vi "Validate VAL SW.vi"() -> ()   [LabVIEW 2023, in "GUI.lvlib" / "Diagnostic.lvlib" / "VAL_SW_Testing.lvlib"]
uses:
  VAL_SW_Testing.lvlib
  HardwareAbstractionLayer_LVOOP/CAN/CAN Lib/CAN_class/Ctrls/CAN Init Ctrl.ctl
  <vilib>/xnet/xnet.llb/XNET Control Scope.ctl
  Ctrls/refresh.ctl
  Ctrls/stop.ctl
  Ctrls/File Paths.ctl
  HardwareAbstractionLayer_LVOOP/CAN/CAN Application Protocols/STP Protocol_class/Ctrls/STP CMD.ctl
  Ctrls/fwd.ctl
  Ctrls/refresh_sqr.ctl
  Ctrls/start.ctl
  HardwareAbstractionLayer_LVOOP/CAN/CAN Lib/Control/CAN Table.ctl
  HardwareAbstractionLayer_LVOOP/CAN/CAN Application Protocols/STP Protocol_class/Ctrls/STP Input Data.ctl
  HardwareAbstractionLayer_LVOOP/Database/SQL Public VI/Control/DB Options.ctl
  <vilib>/Utility/file.llb/Write Delimited Spreadsheet (string).vi
  <userlib>/_OpenG.lib/appcontrol/appcontrol.llb/openg_application_control.lvlib
  HardwareAbstractionLayer_LVOOP/CAN/CAN Application Protocols/STP Protocol_class/STP Protocol.lvclass
  HardwareAbstractionLayer_LVOOP/Database/Database.lvclass
  HardwareAbstractionLayer_LVOOP/CAN/CAN Lib/CAN_class/CAN.lvclass
  Teststand Steptypes/LTT_TeststandSteptypes.lvlib
  HardwareAbstractionLayer_LVOOP/CAN/CAN Lib/CAN HAL Lib.lvlib
panel:
  in  "Stop Button":T1
  in  "Tab Control":T2(tab)
  out "Response Data VAL SW":u8[](array[numeric]) caption="Data" format="%.0x"
  out "Request Timeout_mode":bool caption="Request Timeout?"
  out "+ve Response_Mode":bool caption="+ve Response?"
  in  "Latest_Irms":T3
  out "Irms":cluster{"Numeric 3":dbl, "Numeric 3":dbl}(knob)={"Numeric 3"=0.0, "Numeric 3"=30.81036768238346} scale=0.15..250.0
  in  "Stop Mode":T1
  out "Time Elapsed(Sec)":dbl format="%#.3g"
  in  "Start Mode":T4
  in  "Select Mode":u16(ring)=10 items=["Mode 1: eDCU ON / eMOTOR OFF"=1, "Mode 2: WMTC Pattern 1"=2, "Mode 3: WMTC Pattern 2"=3, "Mode 4: WMTC Pattern 3"=4, "Mode 5: WMTC Pattern 4"=5, "Mode 6: WMTC Pattern 5"=6, "Mode 7: WMTC Pattern 6"=7, "Mode 8: Worst case 1&3"=8, "Mode 9: Full power"=9, " Mode 10: Peak power (Worst case 1)"=10, "Mode 11 : Acceleration (Worst case 3)"=11, "Mode 12 : 1A RMS Continuous"=12, "Mode 13 : 5A RMS Continuous"=13, "Mode 14 : 70A RMS Continuous"=14]
  in  "VAL_Version":T3
  in  "TSW_Version":T3
  out "VAL SW Version":string
  out "TSW Version":string
  in  "Export":bool
  out "Request Timeout? Frame":bool caption="Request Timeout?"
  out "+ve Response? Frame":bool caption="+ve Response?"
  in  "Data Source":enum16{"CSV File", "CAN"}(ring)=enum."CAN"
  out "Datasize(Bytes)":i32
  out "Frame Data":u8[](array[numeric])
  in  "Frame Type":enum16{"FE Frame", "FF Frame"}(ring)
  in  "FE FF Refresh":T5
  in  "Raw_Data?":bool
  in  "Frame Detail":i32(listbox)
  out "Request Timeout?":bool
  out "ResponseData(ASCII)":string
  in  "Send CMD":T6
  out "+ve Response?":bool
  out "Response Data":u8[](array[numeric]) format="%.0x"
  in  "Write Data":u8[](array[numeric]) format="%.0x"
  in  "CMD":T7=130 items=["TSW_VERSION(130)"=130, "WAIT_EVENT(132)"=132, "SEQUENCER(133)"=133, "TSW_RESET(150)"=150, "CONFIG_ECU(151)"=151, "TEST_CORE (152)"=152, "TEST_WATCHDOG (153)"=153, "TEST_MONITORING (154)"=154, "READ_MEMORY (162)"=162, "WRITE_ERASE_MEMORY (164)"=164, "COMM_EXTERNAL (190)"=190, "COMM_INTERNAL (195)"=195, "GET_ANALOG_INPUT (210)"=210, "GET_DIGITAL_INPUT (211)"=211, "GET_FREQUENCY_INPUT (212)"=212, "TEST_INPUT_STRUCTURE (214)"=214, "GENERATE_OUTPUT_SIGNAL (220)"=220, "GENERATE_SYNCHRONIZED_OUTPUT_SIGNALS (221)"=221, "eDCU_Specific (250)"=250]
  in  "Echo?":bool
  in  "Log CAN Data":bool=TRUE
  in  "Timeout(Sec)":dbl=5.0
  in  "Config File Path":T8
  in  "CAN Init Data":T9={"XNET Interface"="CAN3", "Baud Rate"=1000000, "CAN:Termination"=0, "Echo Transmit?"=FALSE, "scope (normal)"=0} {"scope (normal)" items=["Normal", "Session Only", "Interface Only", "Session Only Blocking"]; "CAN:Termination" items=["Off", "On"]; "Baud Rate" format="%.0p"}
  in  "XNET Interface":refnum<k21>="CAN2"
  in  "CAN View Table":T11=-1
  # "Latest RMS Current(Amps)"
  # "SW Version"
  # "VAL Modes"
  # "Min"
  # "Max"
  # "Response"
  # "Request"
  # "Response"
  # "CAN Config"
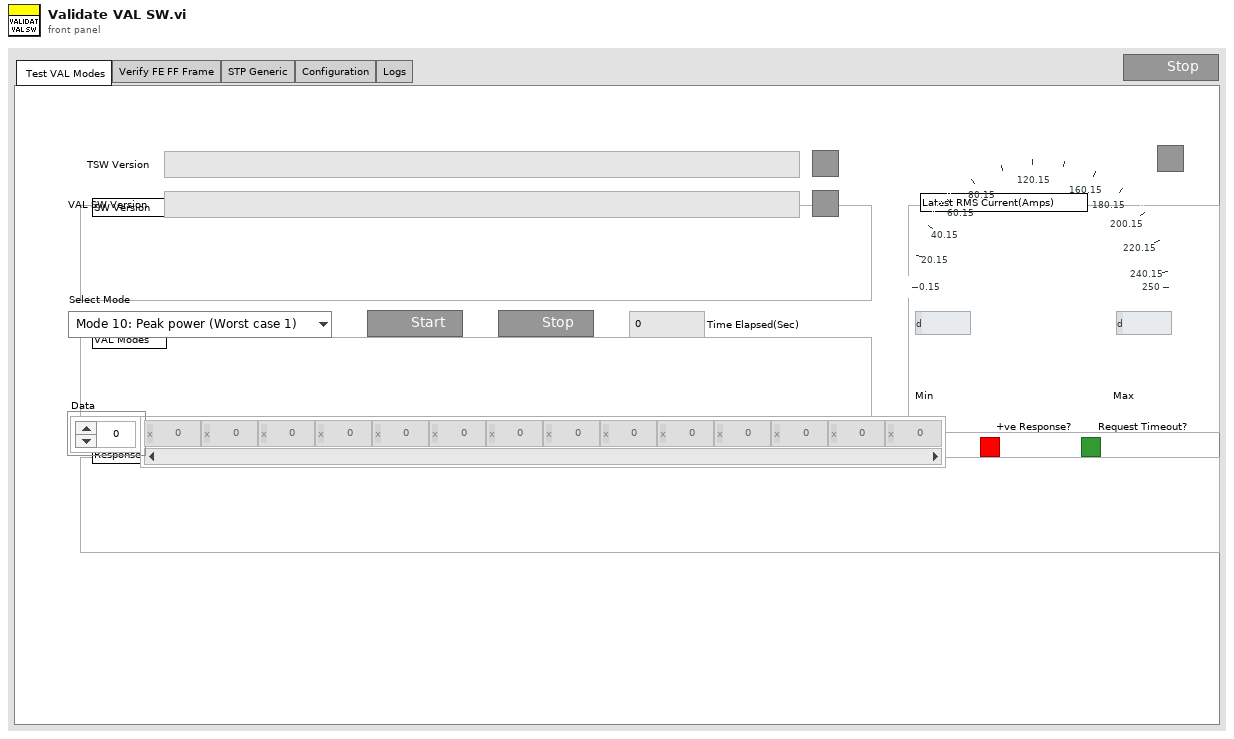
[diagram p1: front panel]
types:
  T1 = typedef "GUI.lvlib/Diagnostic.lvlib/VAL_SW_Testing.lvlib/stop.ctl" = bool
  T2 = enum32{" Test VAL Modes", "Verify FE FF Frame", "STP Generic", "Configuration", "Logs"}
  T3 = typedef "GUI.lvlib/Diagnostic.lvlib/VAL_SW_Testing.lvlib/refresh_sqr.ctl" = bool
  T4 = typedef "GUI.lvlib/Diagnostic.lvlib/VAL_SW_Testing.lvlib/start.ctl" = bool
  T5 = typedef "GUI.lvlib/Diagnostic.lvlib/VAL_SW_Testing.lvlib/refresh.ctl" = bool
  T6 = typedef "GUI.lvlib/Diagnostic.lvlib/VAL_SW_Testing.lvlib/fwd.ctl" = bool
  T7 = typedef "HardwareAbstractionLayer_LVOOP.lvlib/CAN Application Protocols Lib.lvlib/STP Protocol.lvclass/STP CMD.ctl" = u8
  T8 = typedef "GUI.lvlib/Diagnostic.lvlib/VAL_SW_Testing.lvlib/File Paths.ctl" = cluster{"FE_FF_Data File":path, "FE_Frame_Details_File":path, "FF_Frame_Details_File":path}
  T9 = typedef "HardwareAbstractionLayer_LVOOP.lvlib/CAN HAL Lib.lvlib/CAN.lvclass/CAN Init Ctrl.ctl" = cluster{"XNET Interface":refnum<k21>, "Baud Rate":u64, "CAN:Termination":u32, "Echo Transmit?":bool, "scope (normal)":T10}
  T10 = typedef "XNET Control Scope.ctl" = u32
  T11 = typedef "HardwareAbstractionLayer_LVOOP.lvlib/CAN HAL Lib.lvlib/CAN Table.ctl" = i32
  T12 = typedef "HardwareAbstractionLayer_LVOOP.lvlib/Database.lvclass/DB Options.ctl" = enum16{"Init", "Select Data", "Insert Data", "Update Data", "Delete Data", "Execute Query", "Create Schema", "Create Table", "List Tables", "List Columns", "Close"}
  T13 = typedef "HardwareAbstractionLayer_LVOOP.lvlib/CAN Application Protocols Lib.lvlib/STP Protocol.lvclass/STP Input Data.ctl" = cluster{"TxID":u32, "RxID":u32, "CMD":T7, "RQ Data":u8[], "+veResponseCode":u8, "ResponseTimeout (S)":dbl}
  T14 = enum16{"StartTimer", "ReadTimer", "StopTimer", "Init"}
  T15 = enum32{" Test VAL Modes", "Verify FE FF Frame", "STP Generic", "Configuration"}
  T16 = cluster{"Data Source":enum16{"CSV File", "CAN"}, "Frame Type":enum16{"FE Frame", "FF Frame"}, "Raw_Data?":bool, "Config File Path":T8, "CAN Init Data":T9, "ResponseTimeout (S)":dbl}
  T17 = typedef "HardwareAbstractionLayer_LVOOP.lvlib/CAN Application Protocols Lib.lvlib/STP Protocol.lvclass/STP Output Data.ctl" = cluster{"ResponseData":u8[], "ResponseData(ASCII)":string, "PositiveResponse?":bool, "STP Error":T18}
  T18 = typedef "HardwareAbstractionLayer_LVOOP.lvlib/CAN Application Protocols Lib.lvlib/STP Protocol.lvclass/STP Error Cluster.ctl" = cluster{"Status":bool, "Code":u8, "Error":string, "Description":string}
  T19 = cluster{"Frame Data":u8[], "Raw Data":u64[], "Signal Values":string[], "Datasize(Bytes)":i32}
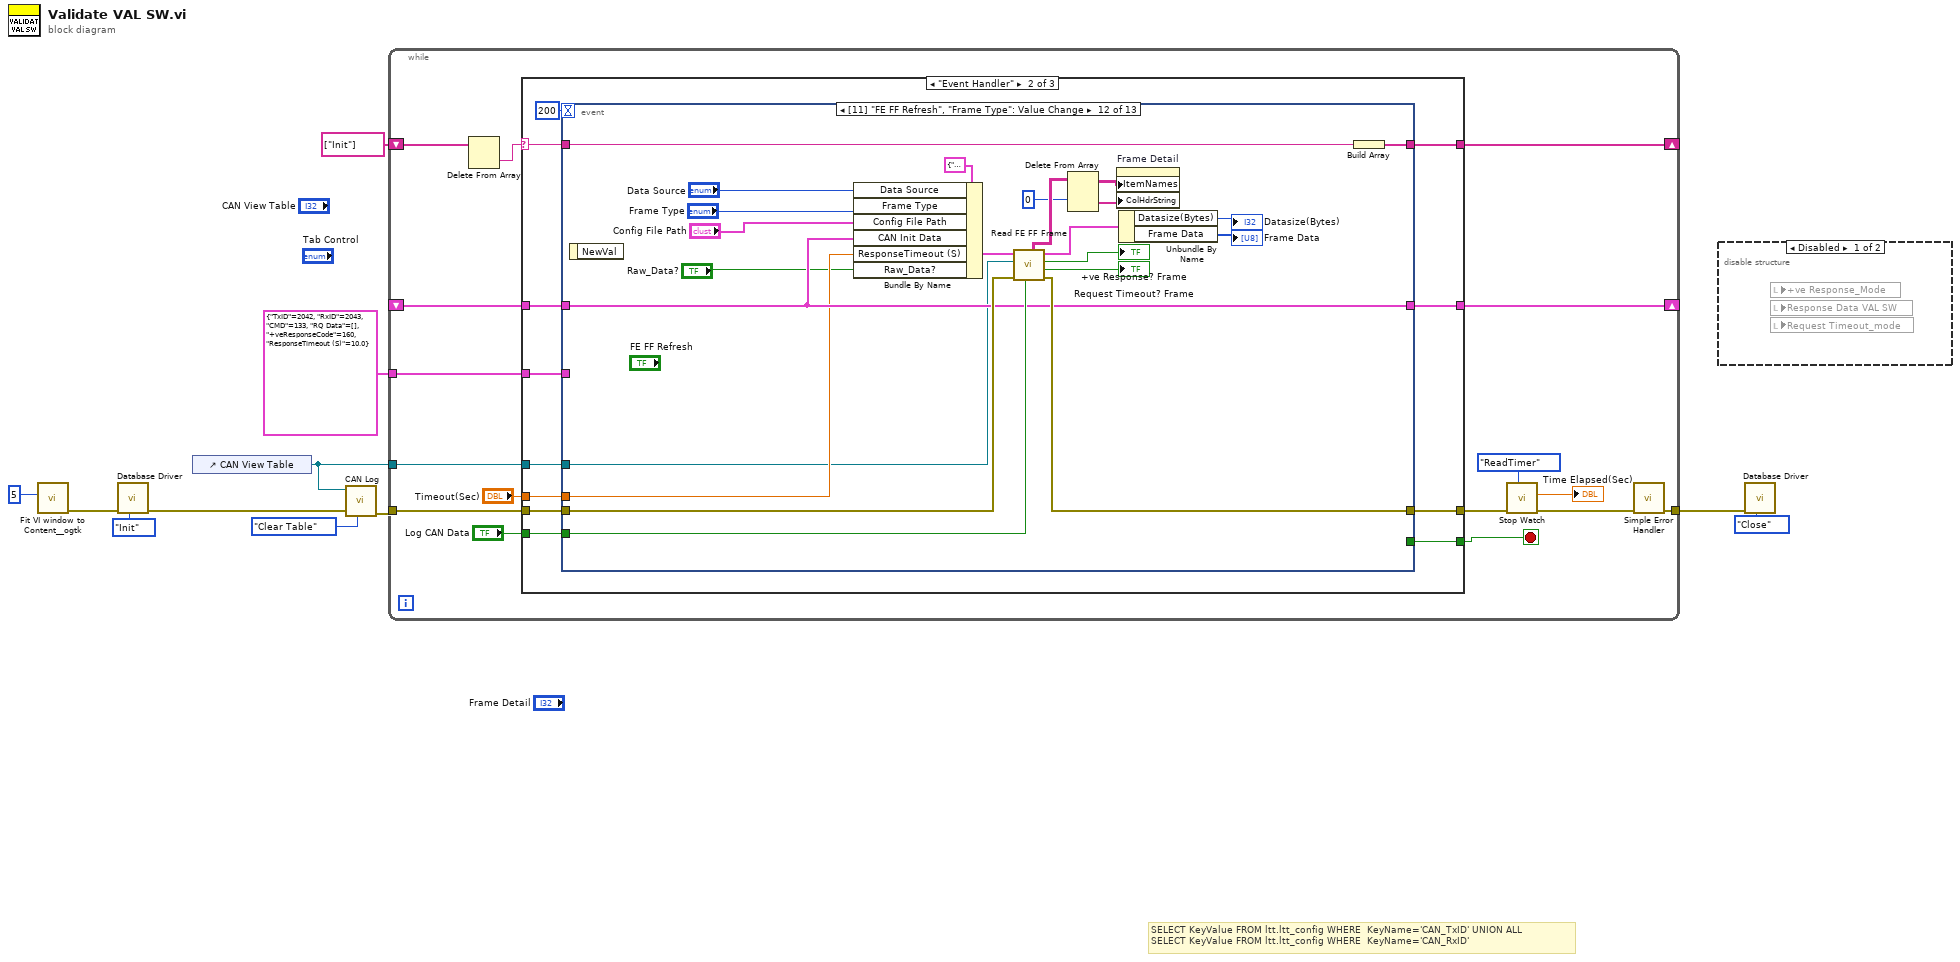
[diagram p0: block diagram]
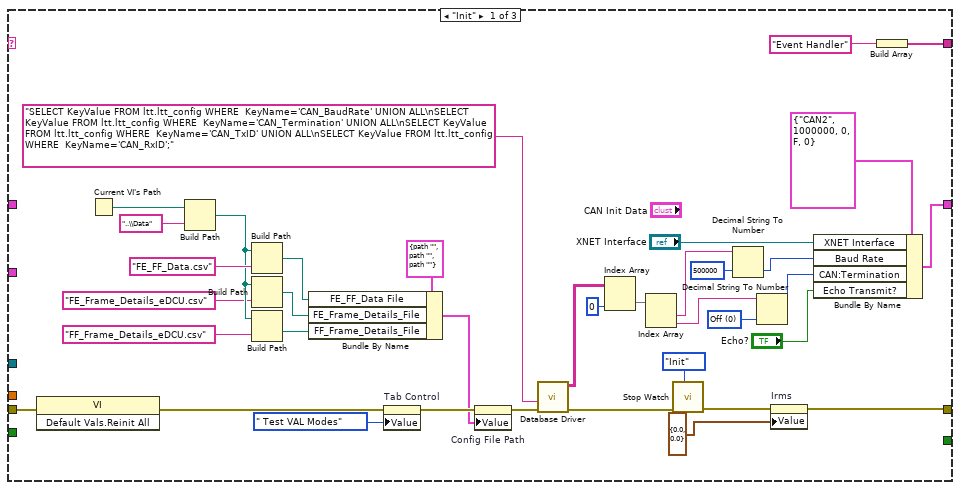
[diagram p3: hidden frame]
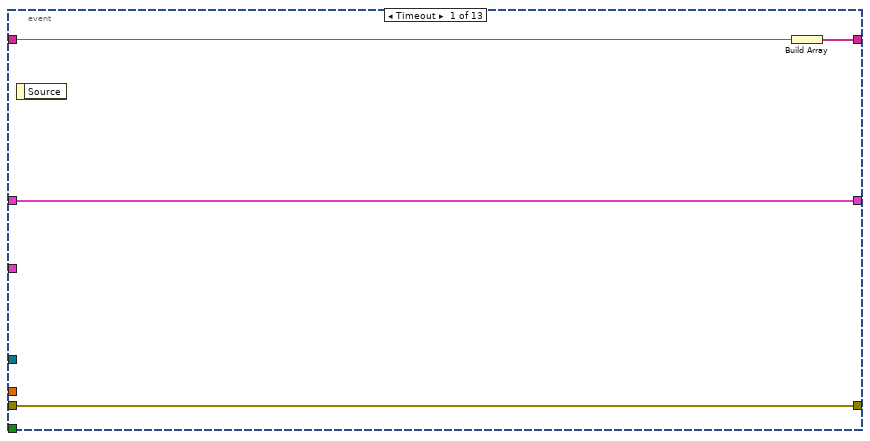
[diagram p4: hidden frame]
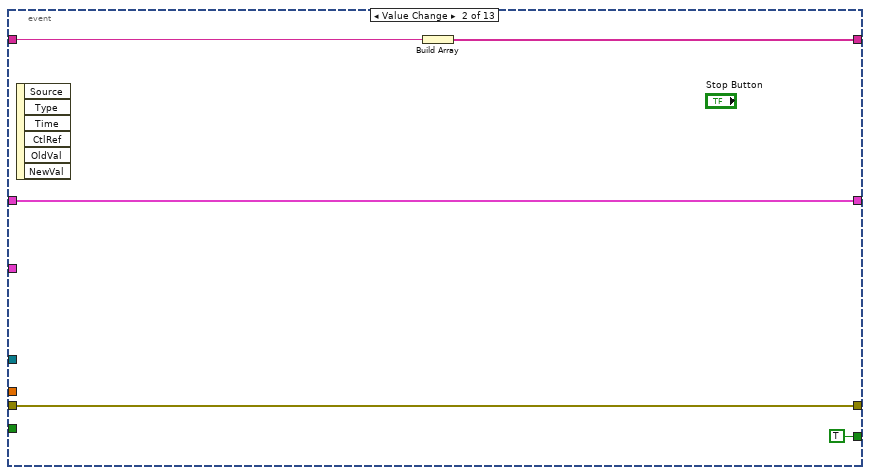
[diagram p5: hidden frame]
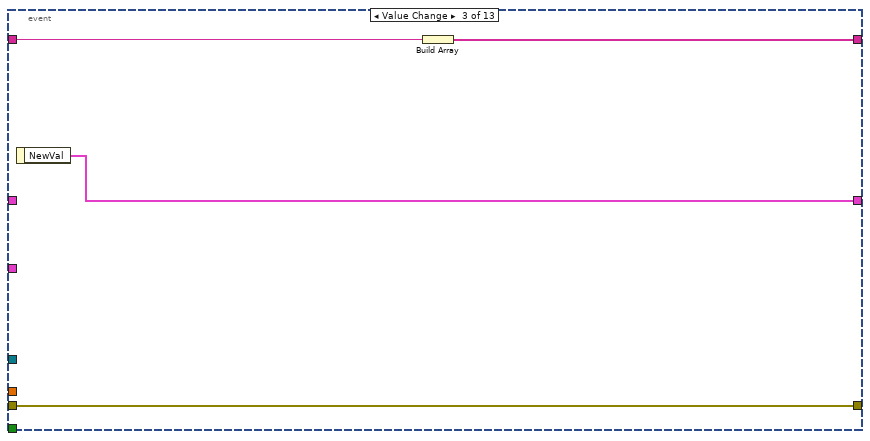
[diagram p6: hidden frame]
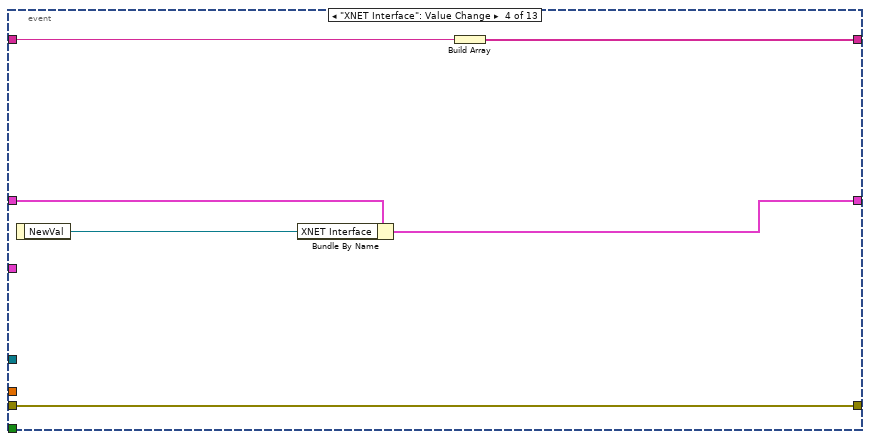
[diagram p7: hidden frame]
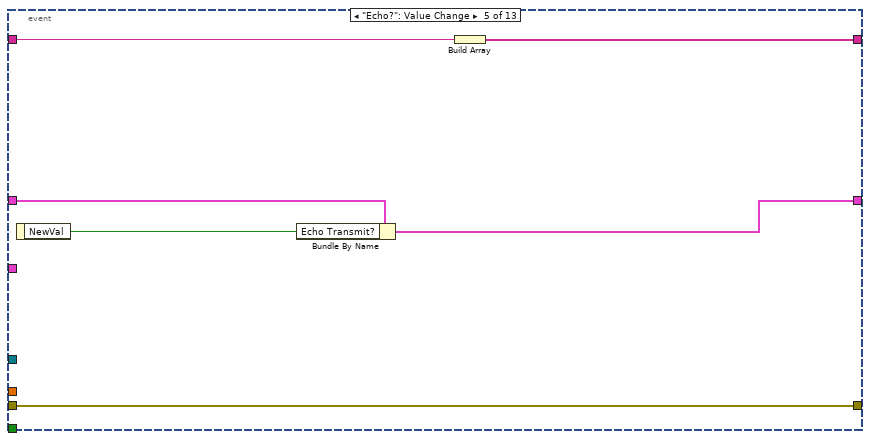
[diagram p8: hidden frame]
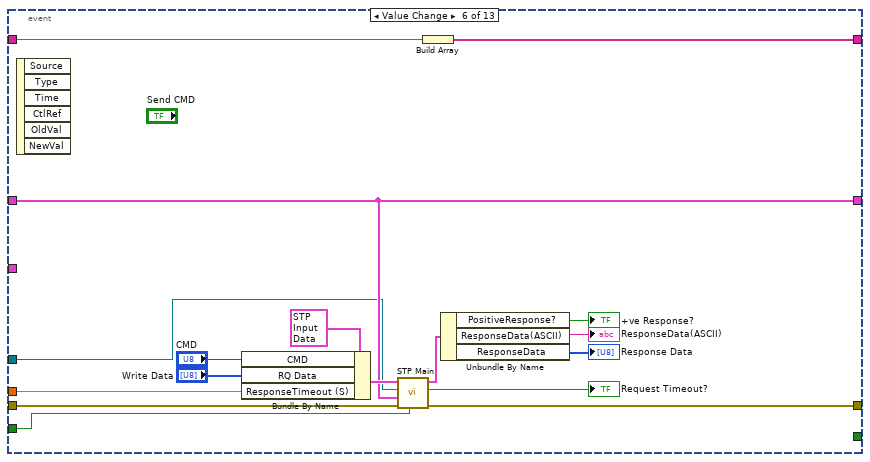
[diagram p9: hidden frame]
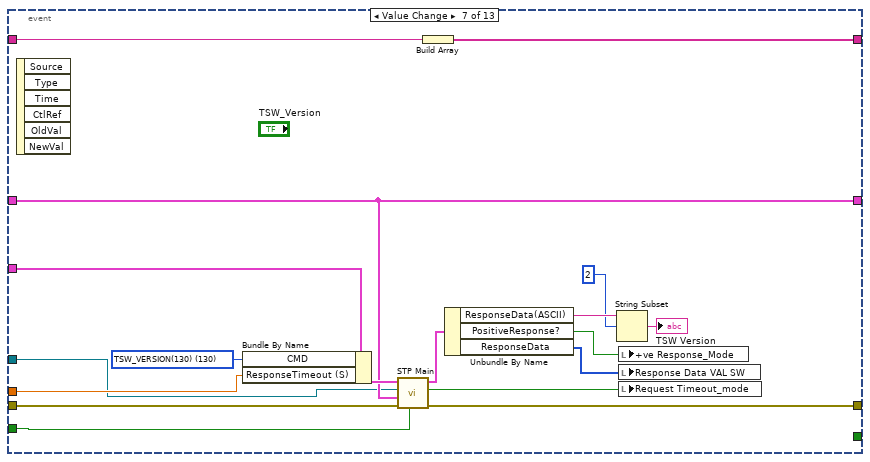
[diagram p10: hidden frame]
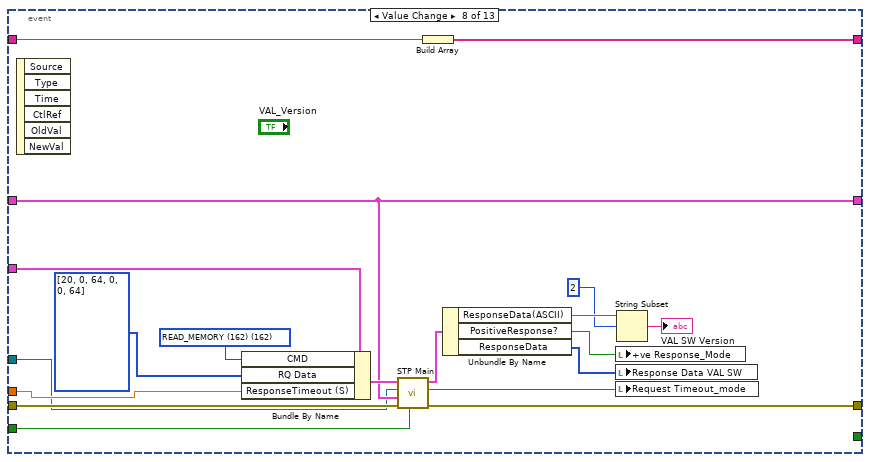
[diagram p11: hidden frame]
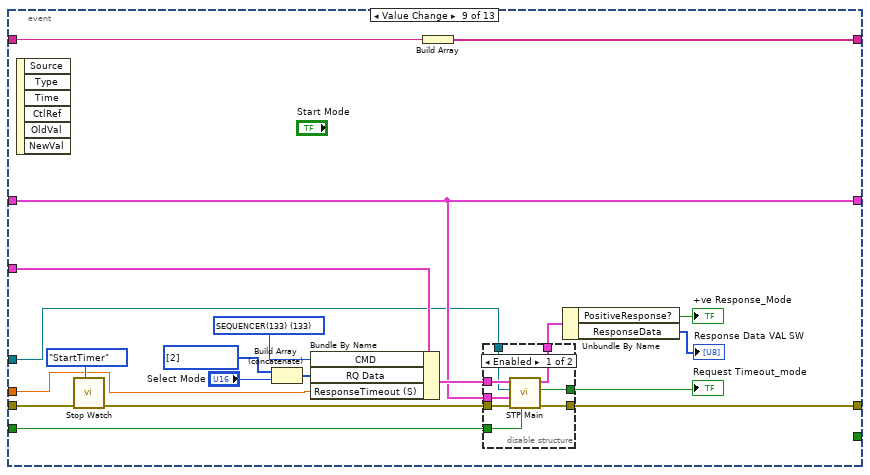
[diagram p12: hidden frame]
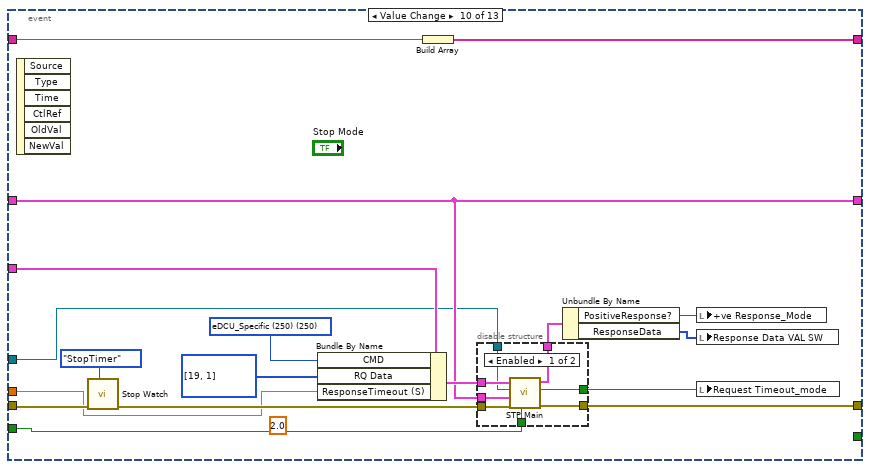
[diagram p14: hidden frame]
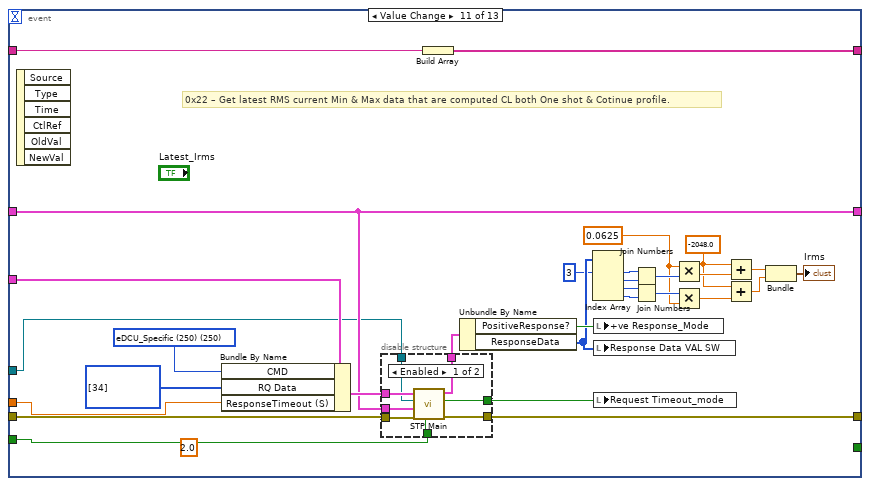
[diagram p16: hidden frame]
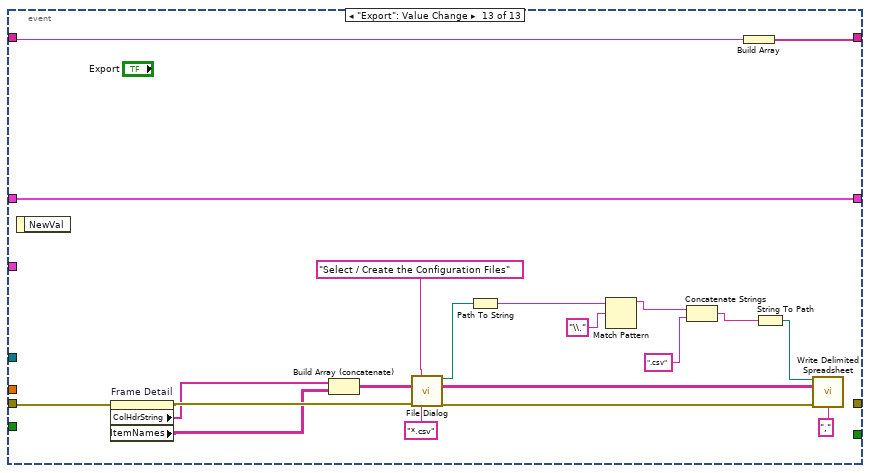
[diagram p18: hidden frame]
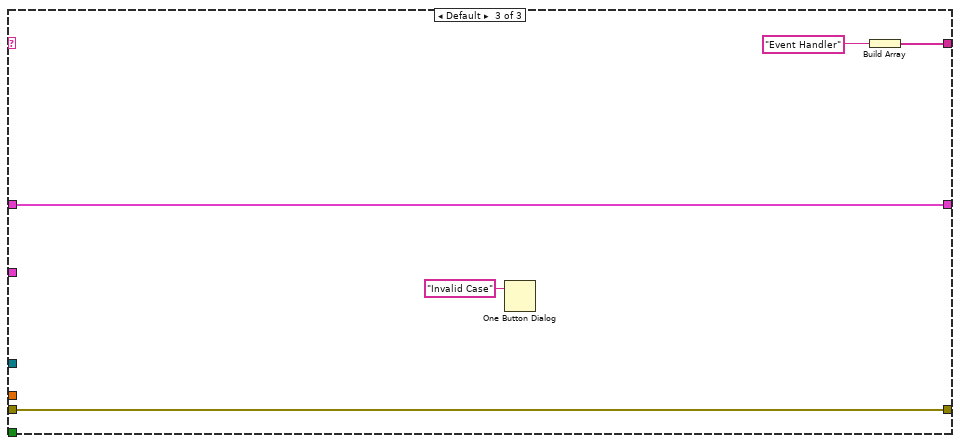
[diagram p19: hidden frame]
diagram:
  # "SELECT KeyValue FROM ltt.ltt_config WHERE  KeyName='CAN_TxID' UNION ALL\nSELECT KeyValue FROM ltt.ltt_config WHERE  KeyName='CAN_RxID'"
  n1 = call <userlib>:"Fit VI window to Content__ogtk.vi"("border spacing (2 px)"=5) -> ("error out"=w7:errorcluster)  [unwired: 5 in, 1 out]
  n2 = call "Database Driver.vi"("Options"=DB_Options."Init", "error in"=w7) -> ("error out"=w2:errorcluster)  [unwired: 6 in, 3 out]
  n3 = control-ref of="CAN View Table"() -> (w4:refnum<vi>)
  n4 = call "CAN Log.vi"("Action"=enum16{"Update Table", "Clear Table"}."Clear Table", "error in (no error)"=w2, "CAN View Table"=w4) -> ("error out"=w1:errorcluster)  [unwired: 8 in]
  n5 = while {
    shift-right: [w25] -> _
    shift-left: string[] ["Init"] -> [w27]
    shift-right: [w24] -> _
    shift-left: _ -> [w23]
    tunnel: T13 {"TxID"=2042, "RxID"=2043, "CMD"=133, "RQ Data"=[], "+veResponseCode"=160, "ResponseTimeout (S)"=10.0} ("STP Input Data") -> [w18]
    tunnel: w4 -> [w17]
    tunnel: w1 -> [w22]
    tunnel: [w12] -> w5
    stop <- w14 stop-if-true
    n6 = Delete From Array(array=w27) -> (deleted portion=w26:string)  [unwired: 2 in, 1 out]
    n7 = case shown="\"Event Handler\"" w26 {
      selector: w26 -> [_ w74 _]
      tunnel: [_ w76 _] -> w14
      tunnel: [w64 w75 w293] -> w25
      tunnel: [w30 w71 w291] -> w24
      tunnel: w23 -> [_ w72 w291]
      tunnel: w22 -> [w62 w70 w290]
      tunnel: [w46 w69 w290] -> w21
      tunnel: w18 -> [_ w68 _]
      tunnel: w17 -> [_ w67 _]
      tunnel: "Log CAN Data" -> [_ w66 _]
      tunnel: "Timeout(Sec)" -> [_ w65 _]
      frame "Init" {
        w39 = u32 0 items=["Off", "On"] ("CAN:Termination")
        n8 = invoke class="VI" method="Default Vals.Reinit All"(error in=w62) -> (error out=w61:errorcluster)  [unwired: 2 in, 2 out]
        n9 = Current VI's Path() -> (path=w60:path)
        n10 = Build Path(base path=w60, name or relative path="..\\Data") -> (appended path=w56:path)
        n11 = Build Path(base path=w56, name or relative path="FE_FF_Data.csv") -> (appended path=w53:path)
        n12 = Build Path(base path=w56, name or relative path="FE_Frame_Details_eDCU.csv") -> (appended path=w52:path)
        n13 = Build Path(base path=w56, name or relative path="FF_Frame_Details_eDCU.csv") -> (appended path=w51:path)
        n14 = Bundle By Name(cluster=T8 {"FE_FF_Data File"=path "", "FE_Frame_Details_File"=path "", "FF_Frame_Details_File"=path ""} ("Config File Path"), "FE_FF_Data File"=w53, "FE_Frame_Details_File"=w52, "FF_Frame_Details_File"=w51) -> (w49:T8)
        n15 = property on="Tab Control" class="TabCtl (strict)"(error in=w61, "Value"=T15." Test VAL Modes" ("Tab Control")) -> (error out=w50:errorcluster)  [unwired: 1 in, 1 out]
        n16 = property on="Config File Path" class="Clust (strict)"(error in=w50, "Value"=w49) -> (error out=w35:errorcluster)  [unwired: 1 in, 1 out]
        n17 = call "Database Driver.vi"("error in"=w35, "SQL query"="SELECT KeyValue FROM ltt.ltt_config WHERE  KeyName='CAN_BaudRate' UNION ALL\nSELECT KeyValue FROM ltt.ltt_config WHERE  KeyName='CAN_Termination' UNION ALL\nSELECT KeyValue FROM ltt.ltt_config WHERE  KeyName='CAN_TxID' UNION ALL\nSELECT KeyValue FROM ltt.ltt_config WHERE  KeyName='CAN_RxID';") -> ("error out"=w34:errorcluster, "data"=w42:string[][])  [unwired: 6 in, 2 out]
        n18 = Index Array(array=w42, index (col)=0 ("disabled index (col)")) -> (element=w40:string[])  [unwired: 1 in]
        n19 = Index Array(array=w40) -> (element #1=w43:string, element #2=w41:string)  [unwired: 2 in]
        n20 = call "Stop Watch.vi"("TimerAction(Read)"=T14."Init", "error in (no error)"=w34) -> ("error out"=w47:errorcluster)  [unwired: 8 in, 1 out]
        n21 = Decimal String To Number(string=w43, default (0L)=u64 500000 ("Baud Rate")) -> (number=w33:u64)  [unwired: 1 in, 1 out]
        n22 = Decimal String To Number(string=w41, default (0L)=w39) -> (number=w32:u32)  [unwired: 1 in, 1 out]
        n23 = property on="Irms" class="Knob (strict)"(error in=w47, "Value"=cluster{"Numeric 3":dbl, "Numeric 3":dbl} {"Numeric 3"=0.0, "Numeric 3"=0.0} ("Irms")) -> (error out=w46:errorcluster)  [unwired: 1 in, 1 out]
        n24 = Bundle By Name(cluster=T9 {"XNET Interface"="CAN2", "Baud Rate"=1000000, "CAN:Termination"=0, "Echo Transmit?"=FALSE, "scope (normal)"=0} ("CAN Init Data"), "XNET Interface"="XNET Interface", "Baud Rate"=w33, "CAN:Termination"=w32, "Echo Transmit?"="Echo?") -> (w30:T9)
        n25 = Build Array("Event Handler") -> (w64:string[])
      }
      frame "Event Handler" {
        n26 = event shown="[11] \"FE FF Refresh\", \"Frame Type\": Value Change" {
          selector: _ -> [_ _ _ _ _ _ _ _ _ _ _ _ _]
          dyn-events: _ -> [_ _ _ _ _ _ _ _ _ _ _ _ _]
          timeout: 200 -> [_ _ _ _ _ _ _ _ _ _ _ _ _]
          tunnel: [_ TRUE _ _ _ _ _ _ _ _ _ _ _] -> w76
          tunnel: [w79 w81 w86 w92 w98 w105 w130 w149 w170 w196 w234 w267 w287] -> w75
          tunnel: w74 -> [w80 w82 w87 w93 w99 w106 w131 w150 w171 w197 w235 w268 w288]
          tunnel: w72 -> [w78 w85 _ w95 w101 w112 w133 w152 w173 w199 w237 w256 w289]
          tunnel: [w78 w85 w89 w91 w97 w112 w133 w152 w173 w199 w237 w256 w289] -> w71
          tunnel: w70 -> [w77 w83 w88 w90 w96 w114 w135 w154 w161 w190 w229 w270 w286]
          tunnel: [w77 w83 w88 w90 w96 w113 w134 w153 w174 w200 w238 w269 _] -> w69
          tunnel: w68 -> [_ _ _ _ _ _ w122 w140 w159 w187 w213 _ _]
          tunnel: w67 -> [_ _ _ _ _ w102 w119 w137 w156 w184 w210 w248 _]
          tunnel: w66 -> [_ _ _ _ _ w104 w121 w139 w158 w186 w212 w262 _]
          tunnel: w65 -> [_ _ _ _ _ w103 w120 w138 w157 w185 w211 w255 _]
          event Timeout {
            n27 = event-data() -> ()  [unwired: 1 in, 1 out]
            n28 = Build Array(w80) -> (w79:string[])
          }
          event Value Change {
            n29 = event-data() -> ()  [unwired: 1 in, 6 out]
            n30 = Build Array(w82) -> (w81:string[])
          }
          event Value Change {
            n31 = event-data() -> ("NewVal"=w89:T9)  [unwired: 1 in]
            n32 = Build Array(w87) -> (w86:string[])
          }
          event "XNET Interface": Value Change {
            n33 = event-data() -> ("NewVal"=w94:refnum<k21>)  [unwired: 1 in]
            n34 = Bundle By Name(cluster=w95, "XNET Interface"=w94) -> (w91:T9)
            n35 = Build Array(w93) -> (w92:string[])
          }
          event "Echo?": Value Change {
            n36 = event-data() -> ("NewVal"=w100:bool)  [unwired: 1 in]
            n37 = Bundle By Name(cluster=w101, "Echo Transmit?"=w100) -> (w97:T9)
            n38 = Build Array(w99) -> (w98:string[])
          }
          event Value Change {
            n39 = event-data() -> ()  [unwired: 1 in, 6 out]
            n40 = Bundle By Name(cluster=T13 {"TxID"=2042, "RxID"=2043, "CMD"=133, "RQ Data"=[2, 254], "+veResponseCode"=160, "ResponseTimeout (S)"=1.0} ("STP Input Data"), "CMD"="CMD", "RQ Data"="Write Data", "ResponseTimeout (S)"=w103) -> (w117:T13)
            n41 = call "STP Main.vi"("Log Data?"=w104, "error in (no error)"=w114, "CAN Init Data"=w112, "CAN View Table"=w102, "STP Input Data"=w117) -> ("error out"=w113:errorcluster, "RequestTimeout?"=→"Request Timeout?":bool, "STP Output Data"=w111:T17)  [unwired: 4 in]
            n42 = Build Array(w106) -> (w105:string[])
            n43 = Unbundle By Name(w111) -> ("PositiveResponse?"=→"+ve Response?":bool, "ResponseData(ASCII)"=→"ResponseData(ASCII)":string, "ResponseData"=→"Response Data":u8[])
          }
          event Value Change {
            w129 = T7 130 items=["TSW_VERSION(130)"=130, "WAIT_EVENT(132)"=132, "SEQUENCER(133)"=133, "CONFIG_ECU(151)"=151, "TEST_CORE (152)"=152, "TEST_WATCHDOG (153)"=153, "TEST_MONITORING (154)"=154, "READ_MEMORY (162)"=162, "WRITE_ERASE_MEMORY (164)"=164, "COMM_EXTERNAL (190)"=190, "COMM_INTERNAL (195)"=195, "GET_ANALOG_INPUT (210)"=210, "GET_DIGITAL_INPUT (211)"=211, "GET_FREQUENCY_INPUT (212)"=212, "TEST_INPUT_STRUCTURE (214)"=214, "GENERATE_OUTPUT_SIGNAL (220)"=220, "GENERATE_SYNCHRONIZED_OUTPUT_SIGNALS (221)"=221, "eDCU_Specific (250)"=250] ("CMD")
            n44 = event-data() -> ()  [unwired: 1 in, 6 out]
            n45 = Bundle By Name(cluster=w122, "CMD"=w129, "ResponseTimeout (S)"=w120) -> (w136:T13)
            n46 = call "STP Main.vi"("Log Data?"=w121, "error in (no error)"=w135, "CAN Init Data"=w133, "CAN View Table"=w119, "STP Input Data"=w136) -> ("error out"=w134:errorcluster, "RequestTimeout?"=w123:bool, "STP Output Data"=w132:T17)  [unwired: 4 in]
            n47 = Build Array(w131) -> (w130:string[])
            n48 = Unbundle By Name(w132) -> ("ResponseData(ASCII)"=w127:string, "PositiveResponse?"=w125:bool, "ResponseData"=w124:u8[])
            n49 = String Subset(string=w127, offset (0)=2) -> (substring=→"TSW Version":string)  [unwired: 1 in]
            n50 = local write "+ve Response_Mode"(w125) -> ()
            n51 = local write "Response Data VAL SW"(w124) -> ()
            n52 = local write "Request Timeout_mode"(w123) -> ()
          }
          event Value Change {
            w148 = T7 162 items=["TSW_VERSION(130)"=130, "WAIT_EVENT(132)"=132, "SEQUENCER(133)"=133, "CONFIG_ECU(151)"=151, "TEST_CORE (152)"=152, "TEST_WATCHDOG (153)"=153, "TEST_MONITORING (154)"=154, "READ_MEMORY (162)"=162, "WRITE_ERASE_MEMORY (164)"=164, "COMM_EXTERNAL (190)"=190, "COMM_INTERNAL (195)"=195, "GET_ANALOG_INPUT (210)"=210, "GET_DIGITAL_INPUT (211)"=211, "GET_FREQUENCY_INPUT (212)"=212, "TEST_INPUT_STRUCTURE (214)"=214, "GENERATE_OUTPUT_SIGNAL (220)"=220, "GENERATE_SYNCHRONIZED_OUTPUT_SIGNALS (221)"=221, "eDCU_Specific (250)"=250] ("CMD")
            n53 = event-data() -> ()  [unwired: 1 in, 6 out]
            n54 = Bundle By Name(cluster=w140, "CMD"=w148, "RQ Data"=u8[] [20, 0, 64, 0, 0, 64], "ResponseTimeout (S)"=w138) -> (w155:T13)
            n55 = call "STP Main.vi"("Log Data?"=w139, "error in (no error)"=w154, "CAN Init Data"=w152, "CAN View Table"=w137, "STP Input Data"=w155) -> ("error out"=w153:errorcluster, "RequestTimeout?"=w143:bool, "STP Output Data"=w151:T17)  [unwired: 4 in]
            n56 = Build Array(w150) -> (w149:string[])
            n57 = Unbundle By Name(w151) -> ("ResponseData(ASCII)"=w147:string, "PositiveResponse?"=w142:bool, "ResponseData"=w141:u8[])
            n58 = local write "+ve Response_Mode"(w142) -> ()
            n59 = local write "Response Data VAL SW"(w141) -> ()
            n60 = local write "Request Timeout_mode"(w143) -> ()
            n61 = String Subset(string=w147, offset (0)=2) -> (substring=→"VAL SW Version":string)  [unwired: 1 in]
          }
          event Value Change {
            w169 = T7 133 items=["TSW_VERSION(130)"=130, "WAIT_EVENT(132)"=132, "SEQUENCER(133)"=133, "CONFIG_ECU(151)"=151, "TEST_CORE (152)"=152, "TEST_WATCHDOG (153)"=153, "TEST_MONITORING (154)"=154, "READ_MEMORY (162)"=162, "WRITE_ERASE_MEMORY (164)"=164, "COMM_EXTERNAL (190)"=190, "COMM_INTERNAL (195)"=195, "GET_ANALOG_INPUT (210)"=210, "GET_DIGITAL_INPUT (211)"=211, "GET_FREQUENCY_INPUT (212)"=212, "TEST_INPUT_STRUCTURE (214)"=214, "GENERATE_OUTPUT_SIGNAL (220)"=220, "GENERATE_SYNCHRONIZED_OUTPUT_SIGNALS (221)"=221, "eDCU_Specific (250)"=250] ("CMD")
            n62 = event-data() -> ()  [unwired: 1 in, 6 out]
            n63 = call "Stop Watch.vi"("TimerAction(Read)"=T14."StartTimer", "error in (no error)"=w161) -> ("error out"=w162:errorcluster)  [unwired: 8 in, 1 out]
            n64 = Build Array (concatenate)(u8[] [2] ("RQ Data"), "Select Mode") -> (w164:u16[])
            n65 = Bundle By Name(cluster=w159, "CMD"=w169, "RQ Data"=w164, "ResponseTimeout (S)"=w157) -> (w175:T13)
            n66 = Build Array(w171) -> (w170:string[])
            n67 = disable-structure shown="Enabled" {
              disable-tunnel: w175 -> [w183 _]
              disable-tunnel: w162 -> [w182 _]
              disable-tunnel: [w181 _] -> w174
              disable-tunnel: w173 -> [w180 _]
              disable-tunnel: [w179 _] -> w172
              disable-tunnel: [w178 _] -> w167
              disable-tunnel: w158 -> [w177 _]
              disable-tunnel: w156 -> [w176 _]
              frame Enabled {
                n68 = call "STP Main.vi"("Log Data?"=w177, "error in (no error)"=w182, "CAN Init Data"=w180, "CAN View Table"=w176, "STP Input Data"=w183) -> ("error out"=w181:errorcluster, "RequestTimeout?"=w178:bool, "STP Output Data"=w179:T17)  [unwired: 4 in]
              }
              frame Disabled {
              }
            }
            "Request Timeout_mode" <- w167
            n69 = Unbundle By Name(w172) -> ("PositiveResponse?"=→"+ve Response_Mode":bool, "ResponseData"=→"Response Data VAL SW":u8[])
          }
          event Value Change {
            (unwired) 2.0 ("ResponseTimeout (S)")
            w195 = T7 250 items=["TSW_VERSION(130)"=130, "WAIT_EVENT(132)"=132, "SEQUENCER(133)"=133, "CONFIG_ECU(151)"=151, "TEST_CORE (152)"=152, "TEST_WATCHDOG (153)"=153, "TEST_MONITORING (154)"=154, "READ_MEMORY (162)"=162, "WRITE_ERASE_MEMORY (164)"=164, "COMM_EXTERNAL (190)"=190, "COMM_INTERNAL (195)"=195, "GET_ANALOG_INPUT (210)"=210, "GET_DIGITAL_INPUT (211)"=211, "GET_FREQUENCY_INPUT (212)"=212, "TEST_INPUT_STRUCTURE (214)"=214, "GENERATE_OUTPUT_SIGNAL (220)"=220, "GENERATE_SYNCHRONIZED_OUTPUT_SIGNALS (221)"=221, "eDCU_Specific (250)"=250] ("CMD")
            n70 = event-data() -> ()  [unwired: 1 in, 6 out]
            n71 = call "Stop Watch.vi"("TimerAction(Read)"=T14."StopTimer", "error in (no error)"=w190) -> ("error out"=w189:errorcluster)  [unwired: 8 in, 1 out]
            n72 = Bundle By Name(cluster=w187, "CMD"=w195, "RQ Data"=u8[] [19, 1], "ResponseTimeout (S)"=w185) -> (w201:T13)
            n73 = Build Array(w197) -> (w196:string[])
            n74 = disable-structure shown="Enabled" {
              disable-tunnel: w201 -> [w209 _]
              disable-tunnel: w189 -> [w208 _]
              disable-tunnel: [w207 _] -> w200
              disable-tunnel: w199 -> [w206 _]
              disable-tunnel: [w205 _] -> w198
              disable-tunnel: [w204 _] -> w192
              disable-tunnel: w186 -> [w203 _]
              disable-tunnel: w184 -> [w202 _]
              frame Enabled {
                n75 = call "STP Main.vi"("Log Data?"=w203, "error in (no error)"=w208, "CAN Init Data"=w206, "CAN View Table"=w202, "STP Input Data"=w209) -> ("error out"=w207:errorcluster, "RequestTimeout?"=w204:bool, "STP Output Data"=w205:T17)  [unwired: 4 in]
              }
              frame Disabled {
              }
            }
            n76 = Unbundle By Name(w198) -> ("PositiveResponse?"=w193:bool, "ResponseData"=w188:u8[])
            n77 = local write "+ve Response_Mode"(w193) -> ()
            n78 = local write "Response Data VAL SW"(w188) -> ()
            n79 = local write "Request Timeout_mode"(w192) -> ()
          }
          event Value Change {
            w217 = -2048.0 ("x")
            w220 = 0.0625
            (unwired) 2.0 ("ResponseTimeout (S)")
            w233 = T7 250 items=["TSW_VERSION(130)"=130, "WAIT_EVENT(132)"=132, "SEQUENCER(133)"=133, "CONFIG_ECU(151)"=151, "TEST_CORE (152)"=152, "TEST_WATCHDOG (153)"=153, "TEST_MONITORING (154)"=154, "READ_MEMORY (162)"=162, "WRITE_ERASE_MEMORY (164)"=164, "COMM_EXTERNAL (190)"=190, "COMM_INTERNAL (195)"=195, "GET_ANALOG_INPUT (210)"=210, "GET_DIGITAL_INPUT (211)"=211, "GET_FREQUENCY_INPUT (212)"=212, "TEST_INPUT_STRUCTURE (214)"=214, "GENERATE_OUTPUT_SIGNAL (220)"=220, "GENERATE_SYNCHRONIZED_OUTPUT_SIGNALS (221)"=221, "eDCU_Specific (250)"=250] ("CMD")
            # "0x22 – Get latest RMS current Min & Max data that are computed CL both One shot & Cotinue profile."
            n80 = event-data() -> ()  [unwired: 1 in, 6 out]
            n81 = Bundle By Name(cluster=w213, "CMD"=w233, "RQ Data"=u8[] [34], "ResponseTimeout (S)"=w211) -> (w239:T13)
            n82 = disable-structure shown="Enabled" {
              disable-tunnel: w239 -> [w247 _]
              disable-tunnel: w229 -> [w246 _]
              disable-tunnel: [w245 _] -> w238
              disable-tunnel: w237 -> [w244 _]
              disable-tunnel: [w243 _] -> w236
              disable-tunnel: [w242 _] -> w230
              disable-tunnel: w212 -> [w241 _]
              disable-tunnel: w210 -> [w240 _]
              frame Enabled {
                n83 = call "STP Main.vi"("Log Data?"=w241, "error in (no error)"=w246, "CAN Init Data"=w244, "CAN View Table"=w240, "STP Input Data"=w247) -> ("error out"=w245:errorcluster, "RequestTimeout?"=w242:bool, "STP Output Data"=w243:T17)  [unwired: 4 in]
              }
              frame Disabled {
              }
            }
            n84 = Build Array(w235) -> (w234:string[])
            n85 = Unbundle By Name(w236) -> ("PositiveResponse?"=w231:bool, "ResponseData"=w228:u8[])
            n86 = Index Array(array=w228, index #1=3 ("index")) -> (element #1=w225:u8, element #2=w226:u8, element #3=w224:u8, element #4=w223:u8)  [unwired: 3 in]
            n87 = local write "+ve Response_Mode"(w231) -> ()
            n88 = local write "Response Data VAL SW"(w228) -> ()
            n89 = local write "Request Timeout_mode"(w230) -> ()
            n90 = Join Numbers(hi=w225, lo=w226) -> ((hi.lo)=w222:u16)
            n91 = Join Numbers(hi=w224, lo=w223) -> ((hi.lo)=w221:u16)
            n92 = Multiply(x=w220, y=w222) -> (x*y=w219:dbl)
            n93 = Multiply(x=w221, y=w220) -> (x*y=w218:dbl)
            n94 = Add(x=w217, y=w219) -> (x+y=w216:dbl)
            n95 = Add(x=w217, y=w218) -> (x+y=w215:dbl)
            n96 = Bundle(w216, w215) -> (→"Irms":cluster{dbl, dbl})  [unwired: 1 in]
          }
          event "Frame Type": Value Change {
            n97 = event-data() -> ()  [unwired: 1 in, 1 out]
            n98 = Bundle By Name(cluster=T16 {"Data Source"=enum."CAN", "Frame Type"=enum."FE Frame", "Raw_Data?"=TRUE, "Config File Path"={"FE_FF_Data File"=path "D:/eDCU LTT/VT LTT Project/Source Code/GUI/Actor/Diagnostic/Instruments UI/CAN/VAL SW Testing/Data/FE_FF_Data.csv", "FE_Frame_Details_File"=path "D:/eDCU LTT/VT LTT Project/Source Code/GUI/Actor/Diagnostic/Instruments UI/CAN/VAL SW Testing/Data/FE_Frame_Details_eDCU.csv", "FF_Frame_Details_File"=path "D:/eDCU LTT/VT LTT Project/Source Code/GUI/Actor/Diagnostic/Instruments UI/CAN/VAL SW Testing/Data/FF_Frame_Details_eDCU.csv"}, "CAN Init Data"={"XNET Interface"="CAN4", "Baud Rate"=1000000, "CAN:Termination"=1, "Echo Transmit?"=FALSE, "scope (normal)"=0}, "ResponseTimeout (S)"=5.0} ("FE_FF_Decoder"), "Data Source"="Data Source", "Frame Type"="Frame Type", "Config File Path"="Config File Path", "CAN Init Data"=w256, "ResponseTimeout (S)"=w255, "Raw_Data?"="Raw_Data?") -> (w260:T16)
            n99 = call "Read FE FF Frame.vi"("Log Data?"=w262, "error in (no error)"=w270, "CAN View Table"=w248, "FE_FF_Decoder"=w260) -> ("error out"=w269:errorcluster, "RequestTimeout?"=→"Request Timeout? Frame":bool, "PositiveResponse?"=→"+ve Response? Frame":bool, "Output Data"=w253:T19, "Frame Detail"=w252:string[][])  [unwired: 3 in]
            n100 = Delete From Array(array=w252, index (row)=0) -> (deleted portion=w249:string[], array with subset deleted=w250:string[][])  [unwired: 2 in]
            n101 = property on="Frame Detail" class="MCListbox (strict)"("ItemNames"=w250, "ColHdrString"=w249) -> ()  [unwired: 2 in, 2 out]
            n102 = Unbundle By Name(w253) -> ("Datasize(Bytes)"=→"Datasize(Bytes)":i32, "Frame Data"=→"Frame Data":u8[])
            n103 = Build Array(w268) -> (w267:string[])
          }
          event "Export": Value Change {
            n104 = event-data() -> ()  [unwired: 1 in, 1 out]
            n105 = property on="Frame Detail" class="MCListbox (strict)"(error in=w286) -> (error out=w273:errorcluster, "ColHdrString"=w272:string[], "ItemNames"=w271:string[][])  [unwired: 1 in, 1 out]
            n106 = Build Array (concatenate)(w272, w271) -> (w285:string[][])
            n107 = call "File Dialog"("prompt"="Select / Create the Configuration Files", "error in"=w273, "pattern (all files)"="*.csv") -> ("selected path"=w283:path, "error out"=w284:errorcluster)  [unwired: 9 in, 2 out]
            n108 = Path To String(path=w283) -> (string=w282:string)
            n109 = Match Pattern(string=w282, regular expression="\\." ("pattern (all files)")) -> (before substring=w281:string)  [unwired: 1 in, 3 out]
            n110 = Concatenate Strings(w281, ".csv" ("string")) -> (w280:string)
            n111 = Build Array(w288) -> (w287:string[])
            n112 = String To Path(string=w280) -> (path=w279:path)
            n113 = call-poly <vilib>:"Write Delimited Spreadsheet.vi"("file path (dialog if empty)"=w279, "2D data"=w285, "error in (no error)"=w284, "delimiter (\\t)"="," ("delimiter (\\t)")) -> ()  [unwired: 10 in, 2 out]
          }
        }
      }
      frame Default {
        n114 = One Button Dialog(message="Invalid Case") -> ()  [unwired: 1 in, 1 out]
        n115 = Build Array("Event Handler") -> (w293:string[])
      }
    }
    n116 = call "Stop Watch.vi"("TimerAction(Read)"=T14."ReadTimer", "error in (no error)"=w21) -> ("error out"=w13:errorcluster, "TimeLapsed(mS)"=→"Time Elapsed(Sec)":dbl)  [unwired: 8 in]
    n117 = call <vilib>:"Simple Error Handler.vi"("error in (no error)"=w13) -> ("error out"=w12:errorcluster)  [unwired: 4 in, 4 out]
  }
  n118 = disable-structure shown="Disabled" {
    frame Disabled {
      n119 = local read "+ve Response_Mode"() -> ()  [unwired: 1 in]
      n120 = local read "Response Data VAL SW"() -> ()  [unwired: 1 in]
      n121 = local read "Request Timeout_mode"() -> ()  [unwired: 1 in]
    }
    frame Enabled {
    }
  }
  n122 = call "Database Driver.vi"("Options"=DB_Options."Close", "error in"=w5) -> ()  [unwired: 6 in, 4 out]
